vi "auto mode.vi"(0 "Autonomous Mode":T1(radio)=enum."Autonomous 1 (Drive)") -> ()   [LabVIEW 2014]
uses:
  <vilib>/Rock Robotics/Network Tables/NT Write Number.vi
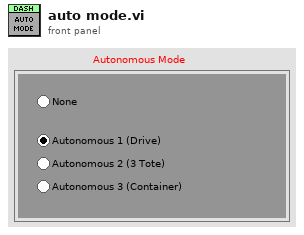
[diagram p1: front panel]
types:
  T1 = enum32{"None", "Autonomous 1 (Drive)", "Autonomous 2 (3 Tote)", "Autonomous 3 (Container)"}
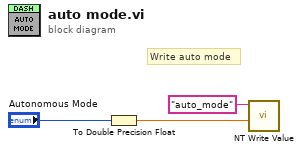
[diagram p0: block diagram]
diagram:
  # "Write auto mode"
  n1 = To Double Precision Float(number="Autonomous Mode") -> (double precision float=w2:dbl)
  n2 = call-poly <vilib>:"NT Write Value.vi"("Numeric"=w2, "Name"="auto_mode") -> ()  [unwired: 9 in, 1 out]
